vi "FinalProject.vi"() -> ()   [LabVIEW 2020]
uses:
  <vilib>/MakerHub/LINX/Public/Sensors/Accelerometer/MPU60X0/DeviceAddresses.ctl
  <vilib>/MakerHub/LINX/Public/Sensors/Accelerometer/MPU60X0/Clock Source.ctl
  <vilib>/MakerHub/LINX/Public/Sensors/Accelerometer/MPU60X0/AccelFullScaleRanges.ctl
  <vilib>/MakerHub/LINX/Public/Sensors/Accelerometer/MPU60X0/GyroFullScaleRanges.ctl
  <vilib>/MakerHub/LINX/Public/Utilities/Open Serial.vi
  <vilib>/MakerHub/LINX/LMH-LINX.lvlib
  <vilib>/MakerHub/LINX/Public/Sensors/Accelerometer/MPU60X0/MPU60X0.lvlib
panel:
  out "?":string
  out "Temp":dbl
  out "Voltage":dbl
  out "Acceleration Data (g)":T1
  out "Gyro  Data (dps)":T1
  out "Acceleration Chart":T1(graph)
  out "Gyro Chart":T1(graph)
  in  "Stop":bool
  in  "VISA resource name":refnum<visa-resource-name>
  out "BPM":dbl
  out "Waveform Chart":dbl(graph)
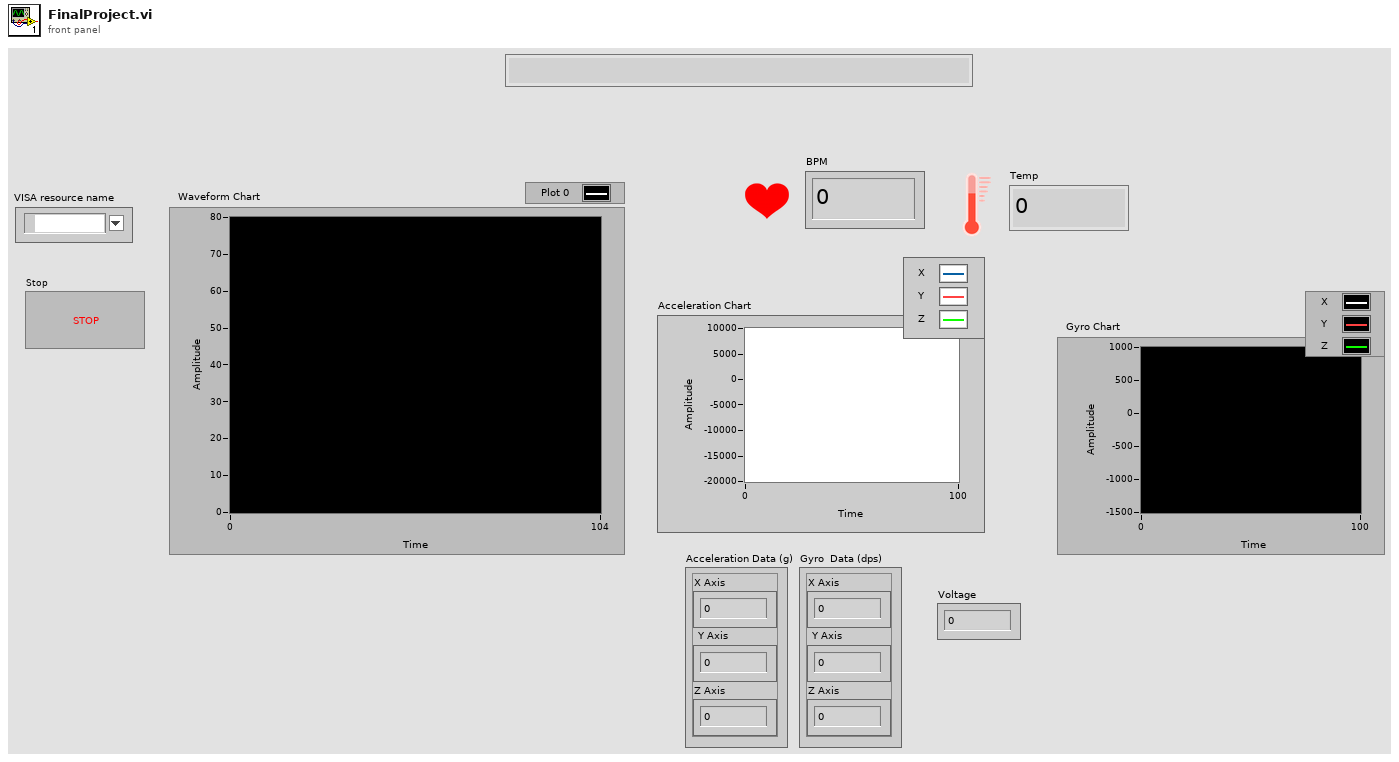
[diagram p1: front panel]
types:
  T1 = cluster{"X Axis":i16, "Y Axis":i16, "Z Axis":i16}
  T2 = typedef "LMH-LINX.lvlib/MPU60X0.lvlib/GyroFullScaleRanges.ctl" = enum8{"±250 °/s", "±500 °/s", "±1000 °/s", "±2000 °/s"}
  T3 = typedef "LMH-LINX.lvlib/MPU60X0.lvlib/AccelFullScaleRanges.ctl" = enum16{"±2g", "±4g", "±8g", "±16g"}
  T4 = typedef "LMH-LINX.lvlib/MPU60X0.lvlib/Clock Source.ctl" = enum8{"Internal 8MHz Osc", "PLL with X Gyro Ref", "PLL with Y Gyro Ref", "PLL with Z Gyro Ref", "PLL with ext 32.768 KHz Ref", "PLL with ext 19.2 MHz Ref", "Reserved", "Hold in reset"}
  T5 = typedef "LMH-LINX.lvlib/MPU60X0.lvlib/DeviceAddresses.ctl" = enum16{"0x68", "0x69"}
  T6 = typedef "LMH-LINX.lvlib/LINX Ref.ctl" = cluster{"IO":T7, "Interface":T8, "LINX Device Config":T9}
  T7 = typedef "LMH-LINX.lvlib/Platform.ctl" = enum16{"Remote", "Local"}
  T8 = typedef "LMH-LINX.lvlib/Interface.ctl" = enum16{"Serial", "TCP"}
  T9 = typedef "LMH-LINX.lvlib/Device.lvlib/LINX Device Config.ctl" = cluster{"Interface":T8, "COM Port":refnum<visa-resource-name>, "TCP Configuration":T10, "Device Family":u8, "Device ID":u8, "Device Name":string, "TCP Ref":refnum<k5>, "Channels":T11}
  T10 = typedef "LMH-LINX.lvlib/Device.lvlib/TCP Config.ctl" = cluster{"IP Address":string, "Port":u16}
  T11 = typedef "LMH-LINX.lvlib/Channels.ctl" = cluster{"DI":u8[], "DO":u8[], "AI":u8[], "AO":u8[], "PWM":u8[], "QE":u8[], "UART":u8[], "I2C 2":u8[], "SPI":u8[], "CAN":u8[], "Servo":u8[], "AI Ref (V)":dbl, "AI Resolution (Bits)":u8, "AO Ref (V)":dbl, "AO Resolution (Bits)":u8}
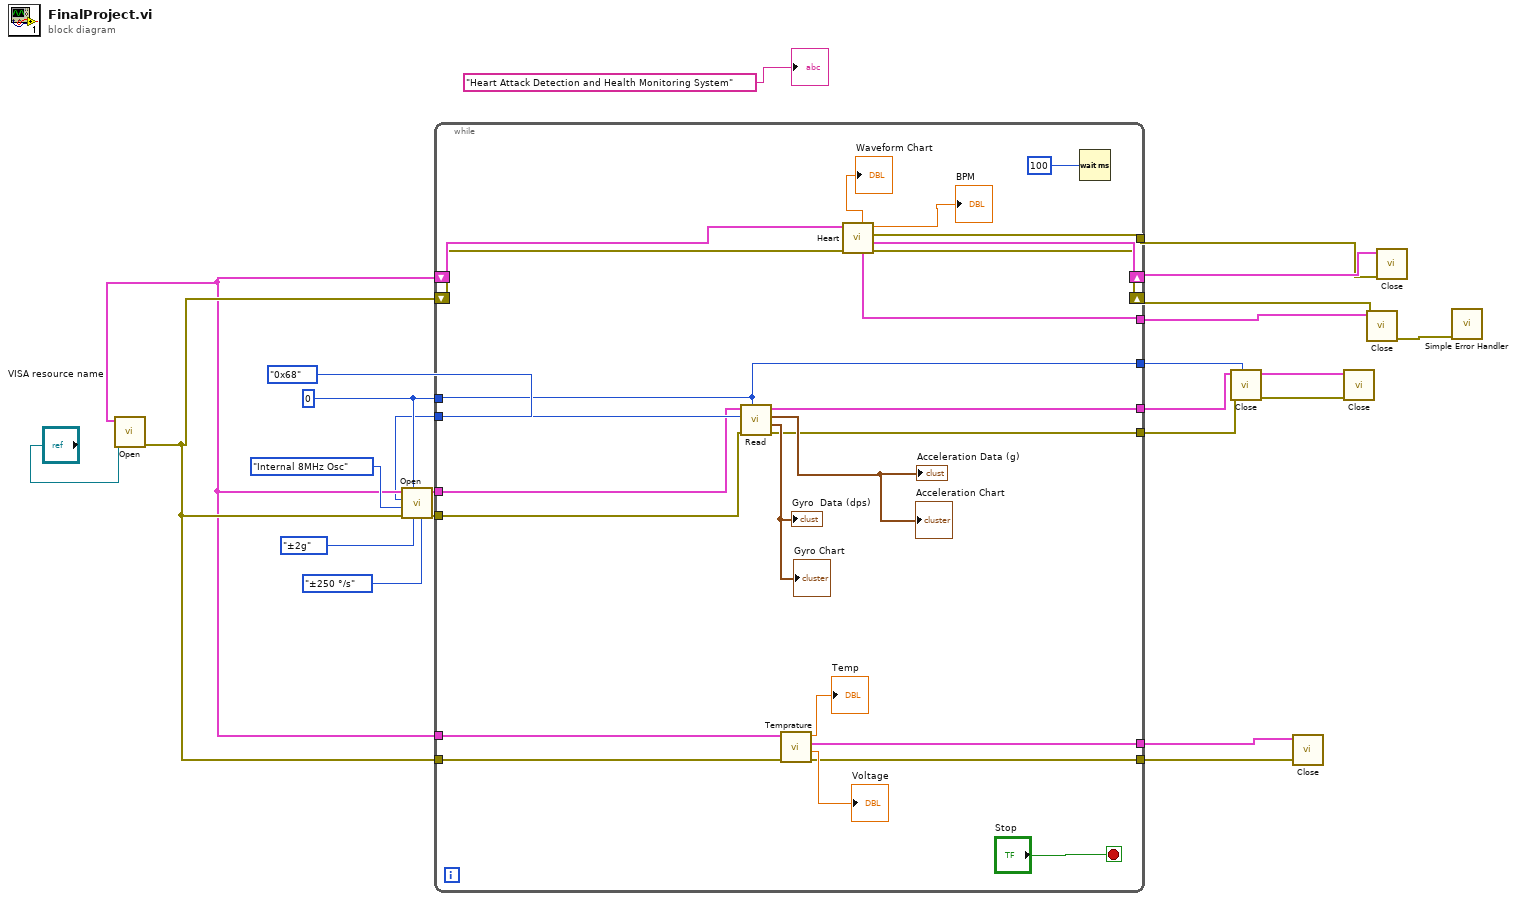
[diagram p0: block diagram]
diagram:
  w13 = u8 0 ("I2C Channel")
  w2 = DeviceAddresses."0x68" ("I2C Slave Address")
  n1 = call-poly <vilib>:"Open.vi"("Serial Port"="VISA resource name") -> ("Error Out"=w8:errorcluster, "LINX Resource"=w7:T6)  [unwired: 8 in, 1 out]
  n2 = call <vilib>:"Open.vi"("Gyro Full Scale Range"=GyroFullScaleRanges."±250 °/s", "Accel Full Scale Range"=AccelFullScaleRanges."±2g", "I2C Channel"=w13, "Error In"=w8, "Clock Source"=Clock_Source."Internal 8MHz Osc", "I2C Slave Address"=w2, "LINX Resource"=w7) -> ("Error Out"=w9:errorcluster, "LINX Resource"=w10:T6)  [unwired: 3 in]
  n3 = while {
    tunnel: [w44] -> w21
    tunnel: [w42] -> w18
    shift-right: [w45] -> w22
    shift-left: w7 -> [w47]
    shift-right: [w43] -> w19
    shift-left: w8 -> [w46]
    tunnel: w13 -> [w36]
    tunnel: [w36] -> w15
    tunnel: w2 -> [w35]
    tunnel: [w34] -> w12
    tunnel: [w33] -> w11
    tunnel: w10 -> [w32]
    tunnel: w9 -> [w31]
    tunnel: w8 -> [w28]
    tunnel: w7 -> [w27]
    tunnel: [w26] -> w6
    tunnel: [w25] -> w5
    stop <- "Stop" stop-if-true
    n4 = call <vilib>:"Read.vi"("I2C Channel"=w36, "Error In"=w31, "I2C Slave Address"=w35, "LINX Resource"=w32) -> ("Error Out"=w34:errorcluster, "Gyro  Data (dps)"=→"Gyro  Data (dps)" →"Gyro Chart":T1, "Acceleration Data (g)"=→"Acceleration Data (g)" →"Acceleration Chart":T1, "LINX Resource"=w33:T6)  [unwired: 3 in, 1 out]
    n5 = call "Temprature.vi"("error in (no error)"=w28, "LINX Resource in"=w27) -> ("error out"=w25:errorcluster, "Voltage"=→"Voltage":dbl, "LINX Resource out"=w26:T6, "Temp"=→"Temp":dbl)  [unwired: 6 in]
    n6 = call "Heart.vi"("error in (no error)"=w46, "LINX Resource 3"=w47) -> ("error out"=w43:errorcluster, "LINX Resource 2"=w45:T6, "Error Out"=w42:errorcluster, "BPM"=→"BPM":dbl, "LINX Resource"=w44:T6, "Waveform Chart"=→"Waveform Chart":dbl)  [unwired: 4 in]
    n7 = Wait (ms)(milliseconds to wait=u32 100 ("millisecond timer value")) -> ()  [unwired: 1 out]
  }
  n8 = call <vilib>:"Close.vi"("I2C Channel (0)"=w15, "Error In"=w12, "LINX Resource"=w11) -> ("Error Out"=w16:errorcluster, "LINX Resource"=w17:T6)  [unwired: 7 in]
  n9 = call <vilib>:"Close.vi"("Error In"=w5, "LINX Resource"=w6) -> ()  [unwired: 9 in, 1 out]
  n10 = call <vilib>:"Close.vi"("Error In"=w16, "LINX Resource"=w17) -> ()  [unwired: 9 in, 1 out]
  n11 = call <vilib>:"Close.vi"("Error In"=w19, "LINX Resource"=w21) -> ("Error Out"=w20:errorcluster)  [unwired: 9 in]
  n12 = call <vilib>:"Close.vi"("Error In"=w18, "LINX Resource"=w22) -> ()  [unwired: 9 in, 1 out]
  n13 = call <vilib>:"Simple Error Handler.vi"("error in (no error)"=w20) -> ()  [unwired: 4 in, 5 out]
  "?" <- "Heart Attack Detection and Health Monitoring System"
